vi "Procesado_aRMS_BIdirecc_Freq_Energia.vi"(0 "Distancias centrales de las ruedas\n               configuración (m)":dbl[](array[numeric]), 1 "Puntos":sgl[](array[numeric]), 2 "dt RMS 2":dbl, 3 "Parámetros acelerómetros":dbl[](array[numeric]), 4 "Frecuencia de muestreo":dbl, 5 "Distancias generales (m)":dbl[](array[numeric]), 6 "Radios por ejes":dbl[](array[numeric]), 7 "high cutoff freq: fh":dbl=0.45000000000000007 format="%0.2f", 9 "low cutoff freq: fl":dbl=0.12500000000000006 format="%0.4f", 10 "Ejes Procesados":i32, 11 "Distancias\nacelerometros":dbl[](array[numeric]), 13 "Paths_canales_aRMS":path[](array[path])) -> (14 "Max RMS Ruedas":dbl[][](array[numeric]), 15 "Frecuencias de rueda":dbl[][](array[numeric]), 17 "Amplitudes":dbl[][](array[numeric]), 18 "Energía":dbl[][](array[numeric]))   [LabVIEW 2015]
uses:
  <vilib>/Analysis/3filter.llb/Filter Passband Type.ctl
  <vilib>/Analysis/baseanly.llb/Mean (DBL).vi
  <vilib>/Analysis/2dsp.llb/Real FFT.vi
  <vilib>/Analysis/8numeric.llb/1D Numeric Integration.vi
  <vilib>/Analysis/5stat.llb/RMS (DBL).vi
  <vilib>/Analysis/3filter.llb/Butterworth Filter (DBL).vi
  <vilib>/measure/madcrms.llb/Basic Averaged DC-RMS for 1 Chan.vi
  <vilib>/measure/NI_MAPro.lvlib
  <vilib>/Analysis/NI_AALBase.lvlib
  <vilib>/Analysis/NI_AALPro.lvlib
panel:
  out "XY Graph":cluster{dbl, dbl}[](graph)
  out "Array 2":dbl[][](array[numeric])
  out "Array":dbl[][](array[numeric])
  out "Loop Rate (Hz)":dbl
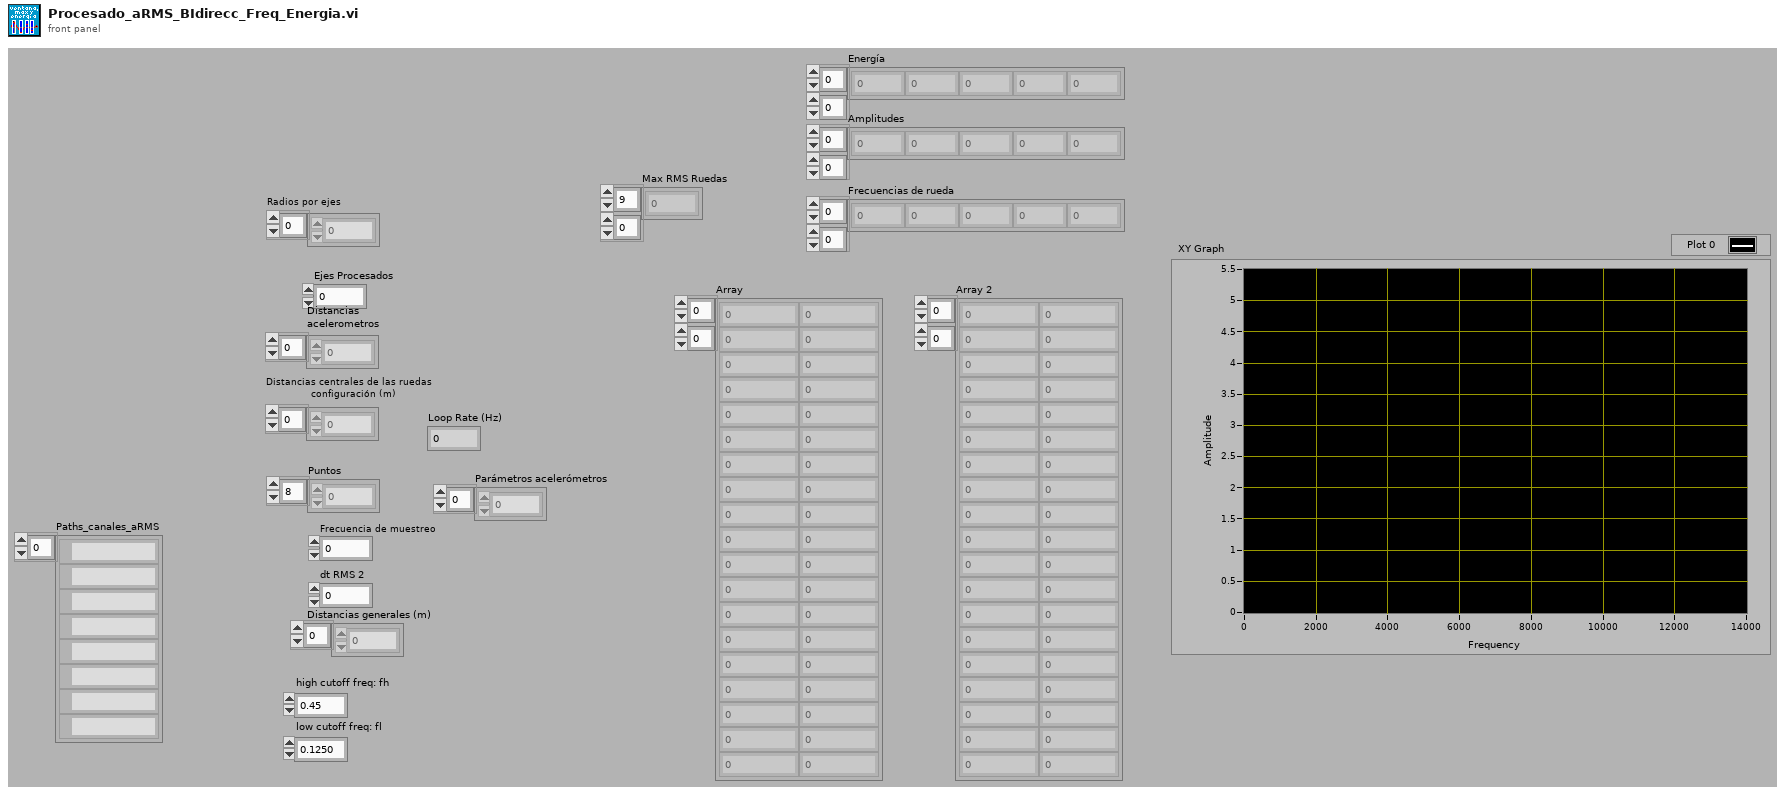
[diagram p1: front panel]
types:
  T1 = typedef "NI_AALBase.lvlib/Filter Passband Type.ctl" = enum32{"Lowpass", "Highpass", "Bandpass", "Bandstop"}
  T2 = enum16{"big-endian, network order", "native, host order", "little-endian"}
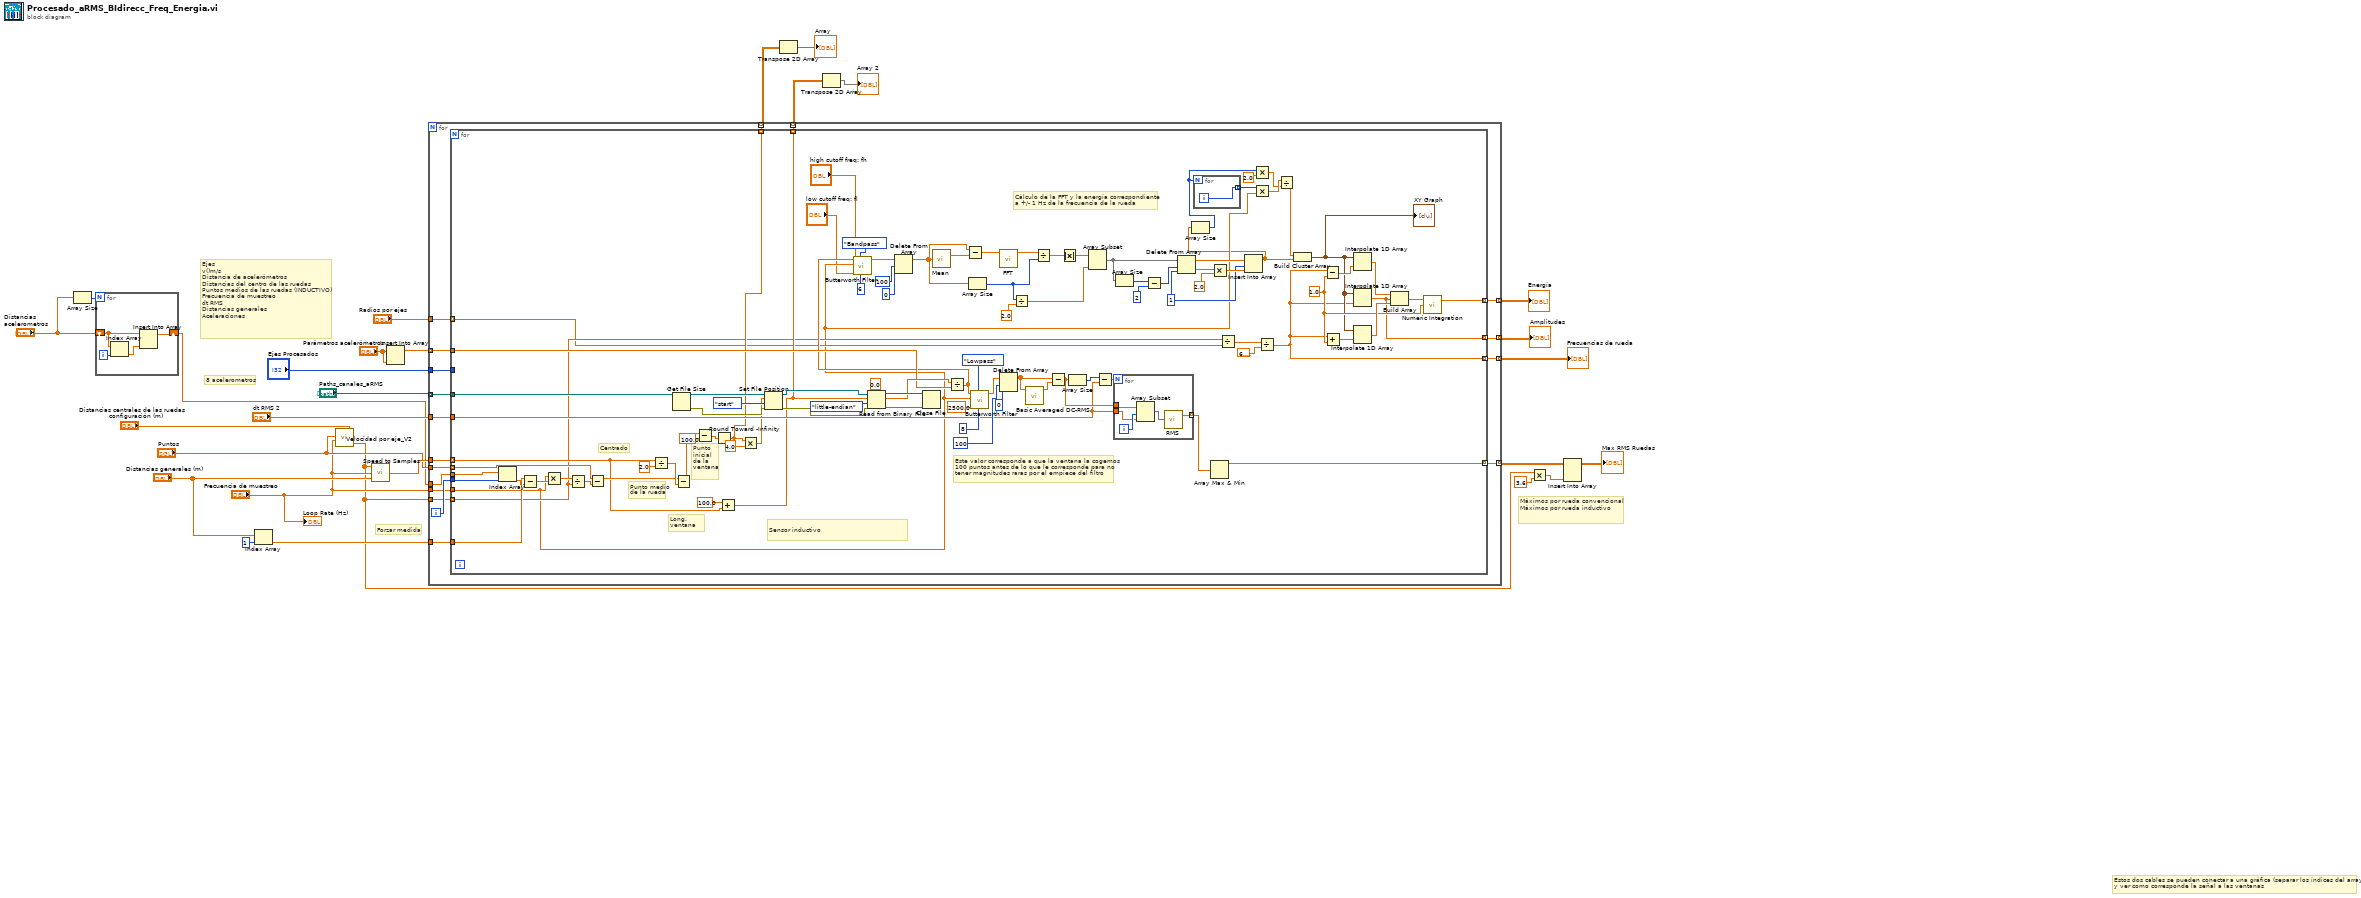
[diagram p0: block diagram]
diagram:
  # "Forzar medida"
  # "8 acelerometros"
  # "Ejes\nv()m/s\nDistancia de acelerómetros\nDistancias del centro de las ruedas\nPuntos medios de las ruedas (INDUCTIVO)\nFrecuencia de muestreo\ndt RMS\nDistancias generales\nAceleraciones"
  # "Máximos por rueda convencional\nMáximos por rueda inductivo"
  # "Estos dos cables se pueden conectar a una gráfica (separar los índices del array)\ny ver como corresponde la señal a las ventanas"
  n1 = Array Size(array="Distancias\nacelerometros") -> (size(s)=w13:i32)
  n2 = for {
    N: w13 -> [_]
    shift-right: [w32] -> w7
    shift-left: "Distancias\nacelerometros" -> [w31]
    i -> [w30]
    n3 = Index Array(array=w31, index=w30) -> (element=w29:dbl)
    n4 = Insert Into Array(array=w31, new element=w29) -> (w32:dbl[])  [unwired: 1 in]
  }
  n5 = Index Array(array="Distancias generales (m)", index=1) -> (element=w6:dbl)
  n6 = call "Velocidad por eje_V2.vi"("Distancias centrales de las ruedas\n               configuración (m)"="Distancias centrales de las ruedas\n               configuración (m)", "Frecuencia de muestreo"="Frecuencia de muestreo", "Puntos centrales de las ruedas\n             inductivo"="Puntos") -> ("Velocidad de eje"=w4:dbl[])  [unwired: 2 in]
  n7 = call "Speed to Samples.vi"("Distancias generales (m)"="Distancias generales (m)", "Loop Rate (Hz)"="Frecuencia de muestreo", "Velocidad de eje(m/s)"=w4) -> ("Longitud de ventana (puntos)"=w28:dbl[])
  n8 = Insert Into Array(array="Parámetros acelerómetros", new element="Parámetros acelerómetros") -> (w18:dbl[])  [unwired: 1 in]
  n9 = for {
    tunnel: w28 -> [w40]
    tunnel: "Puntos" -> [w48]
    tunnel: w4 -> [w45]
    tunnel: w7 -> [w49]
    tunnel: "dt RMS 2" -> [w50]
    tunnel: [w47] -> w24 mode=indexing
    tunnel: "Ejes Procesados" -> [w41]
    tunnel: "Frecuencia de muestreo" -> [w42]
    tunnel: "Paths_canales_aRMS" -> [w44] mode=indexing
    tunnel: w18 -> [w43] mode=indexing
    tunnel: w6 -> [w39]
    tunnel: [w38] -> w8 mode=indexing
    tunnel: [w37] -> w11 mode=indexing
    tunnel: "Radios por ejes" -> [w36]
    tunnel: [w35] -> w3 mode=indexing
    tunnel: [w34] -> w1 mode=indexing
    tunnel: [w33] -> w2 mode=indexing
    i -> [w46]
    n10 = for {
      tunnel: w50 -> [w105]
      tunnel: w49 -> [w143]
      tunnel: w48 -> [w142] mode=indexing
      tunnel: [w141] -> w47 mode=indexing
      tunnel: w46 -> [w140]
      tunnel: w45 -> [w69] mode=indexing
      tunnel: w44 -> [w126]
      tunnel: w43 -> [w134]
      tunnel: w42 -> [w65]
      tunnel: w41 -> [_]
      tunnel: w40 -> [w116] mode=indexing
      tunnel: w39 -> [w103]
      tunnel: [w100] -> w38 mode=indexing
      tunnel: [w99] -> w37 mode=indexing
      tunnel: w36 -> [w68] mode=indexing
      tunnel: [w56] -> w35 mode=indexing
      tunnel: [w53] -> w34 mode=indexing
      tunnel: [w55] -> w33 mode=indexing
      w57 = 1.0
      w77 = 1
      # "Cálculo de la FFT y la energía correspondiente \na +/- 1 Hz de la frecuencia de la rueda"
      # "Este valor corresponde a que la ventana la cogemos\n100 puntos antes de lo que le corresponde para no \ntener magnitudes raras por el empiece del filtro"
      # "Centrado"
      # "Sensor inductivo"
      # "Long.\nventana"
      # "Punto\ninicial\nde la \nventana"
      # "Punto medio\nde la rueda"
      n11 = Index Array(array=w143, index=w140) -> (element=w102:dbl)
      n12 = Subtract(x=w103, y=w102) -> (x-y=w129:dbl)
      n13 = Multiply(x=w65, y=w129) -> (x*y=w131:dbl)
      n14 = Divide(x=w131, y=w69) -> (x/y=w130:dbl)
      n15 = Subtract(x=w142, y=w130) -> (x-y=w119:dbl)
      n16 = Divide(x=w116, y=2.0) -> (x/y=w127:dbl)
      n17 = Get File Size(file=w126) -> (refnum out=w124:refnum<file>, 0:w121:errorcluster)  [unwired: 1 in, 1 out]
      n18 = Subtract(x=w119, y=w127) -> (x-y=w110:dbl)
      n19 = Subtract(x=w110, y=100.0 ("x")) -> (x-y=w118:dbl)
      n20 = Round Toward -Infinity(1:w118) -> (0:w100:dbl)
      n21 = Add(x=100.0, y=w116) -> (x+y=w99:dbl)
      n22 = Multiply(x=w100, y=4.0) -> (x*y=w101:dbl)
      n23 = Set File Position(offset (in bytes) (0)=w101, refnum=w124, from (0:start)=enum16{"start", "end", "current"}."start", error in=w121) -> (refnum out=w122:refnum<file>, error out=w120:errorcluster)
      n24 = Read from Binary File(5:sgl 0.0, 8:w120, 9:T2."little-endian" ("byte order (0:big-endian, network order)"), 10:w99, 11:w122) -> (0:w138:errorcluster, 2:w135:sgl[], 3:w139:refnum<file>)  [unwired: 2 out]
      n25 = Close File(refnum=w139, error in=w138) -> ()  [unwired: 2 out]
      n26 = Divide(x=w135, y=w134) -> (x/y=w97:dbl[])
      n27 = call-poly <vilib>:"Butterworth Filter.vi"("order"=6, "filter type"=Filter_Passband_Type."Bandpass", "low cutoff freq: fl"="low cutoff freq: fl", "high cutoff freq: fh"="high cutoff freq: fh", "sampling freq: fs"=w65, "X"=w97) -> ("Filtered X"=w94:dbl[])  [unwired: 2 in, 1 out]
      n28 = Delete From Array(array=w94, length=100, index=0) -> (array with subset deleted=w75:dbl[])  [unwired: 1 out]
      n29 = call-poly <vilib>:"Mean.vi"("X"=w75) -> ("mean"=w92:dbl)  [unwired: 1 out]
      n30 = Subtract(x=w75, y=w92) -> (x-y=w91:dbl[])
      n31 = Array Size(array=w75) -> (size(s)=w87:i32)
      n32 = call-poly <vilib>:"Butterworth Filter.vi"("order"=8, "filter type"=Filter_Passband_Type."Lowpass", "low cutoff freq: fl"=2500.0, "sampling freq: fs"=w65, "X"=w97) -> ("Filtered X"=w115:dbl[])  [unwired: 3 in, 1 out]
      n33 = call-poly <vilib>:"FFT.vi"("X"=w91) -> ("FFT {X}"=w89:cdb[])  [unwired: 9 in, 1 out]
      n34 = Delete From Array(array=w115, length=100, index=0) -> (array with subset deleted=w114:dbl[])  [unwired: 1 out]
      n35 = Divide(x=w87, y=2.0) -> (x/y=w76:dbl)
      n36 = call-poly <vilib>:"Basic Averaged DC-RMS.vi"("signal in"=w114) -> ("DC value"=w144:dbl)  [unwired: 4 in, 6 out]
      n37 = Divide(x=w89, y=w87) -> (x/y=w90:cdb[])
      n38 = Subtract(x=w114, y=w144) -> (x-y=w108:dbl[])
      n39 = Absolute Value(x=w90) -> (abs(x)=w88:dbl[])
      n40 = Array Size(array=w108) -> (size(s)=w106:i32)
      n41 = Array Subset(array=w88, length=w76) -> (w85:dbl[])  [unwired: 1 in]
      n42 = Subtract(x=w106, y=w105) -> (x-y=w107:dbl)
      n43 = for {
        N: w107 -> [_]
        tunnel: w105 -> [w147]
        tunnel: [w150] -> w104 mode=indexing
        tunnel: w108 -> [w149]
        i -> [w148]
        n44 = Array Subset(array=w149, index=w148, length=w147) -> (w146:dbl[])
        n45 = call-poly <vilib>:"RMS.vi"("X"=w146) -> ("rms value"=w150:dbl)  [unwired: 1 out]
      }
      n46 = Array Size(array=w85) -> (size(s)=w84:i32)
      n47 = Subtract(x=w84, y=2) -> (x-y=w82:i32)
      n48 = Delete From Array(array=w85, length=w82, index=w77) -> (deleted portion=w81:dbl[], array with subset deleted=w78:dbl[])
      n49 = Array Max & Min(array=w104) -> (max value=w141:dbl)  [unwired: 3 out]
      n50 = Multiply(x=w81, y=2.0) -> (x*y=w79:dbl[])
      n51 = Divide(x=w69, y=w68) -> (x/y=w67:dbl)
      n52 = Insert Into Array(array=w78, index=w77, new element=w79) -> (w63:dbl[])
      n53 = Array Size(array=w63) -> (size(s)=w70:i32)
      n54 = for {
        N: w70 -> [_]
        tunnel: [w145] -> w74 mode=indexing
        i -> [w145]
      }
      n55 = Multiply(x=w70, y=2.0) -> (x*y=w71:dbl)
      n56 = Multiply(x=w74, y=w65) -> (x*y=w73:dbl[])
      n57 = Divide(x=w67, y=6.283185307179586) -> (x/y=w53:dbl)
      n58 = Divide(x=w73, y=w71) -> (x/y=w64:dbl[])
      n59 = Build Cluster Array(w64, w63) -> (w54:cluster{dbl, dbl}[])
      "XY Graph" <- w54
      n60 = Subtract(x=w53, y=w57) -> (x-y=w62:dbl)
      n61 = Add(x=w53, y=w57) -> (x+y=w61:dbl)
      n62 = Interpolate 1D Array(1:w62, 2:w54) -> (0:w60:dbl)
      n63 = Interpolate 1D Array(1:w53, 2:w54) -> (0:w55:dbl)
      n64 = Interpolate 1D Array(1:w61, 2:w54) -> (0:w59:dbl)
      n65 = Build Array(w60, w55, w59) -> (w58:dbl[])
      n66 = call-poly <vilib>:"Numeric Integration.vi"("dt"=w57, "Input Array"=w58) -> ("result"=w56:dbl)  [unwired: 1 in, 1 out]
    }
  }
  "Energía" <- w3
  "Amplitudes" <- w2
  "Frecuencias de rueda" <- w1
  n67 = Transpose 2D Array(2D array=w8) -> (transposed array=→"Array":dbl[][])
  n68 = Transpose 2D Array(2D array=w11) -> (transposed array=→"Array 2":dbl[][])
  n69 = Multiply(x=w4, y=3.6) -> (x*y=w21:dbl[])
  n70 = Insert Into Array(array=w24, new element=w21) -> (→"Max RMS Ruedas":dbl[][])  [unwired: 2 in]
  "Loop Rate (Hz)" <- "Frecuencia de muestreo"
